vi "ramp.vi"(2 "start /single":dbl=1200.0, 3 "Number of points":i32=2, 4 "Scan type":T1(ring)=enum."Logarithmic ramp", 5 "chosen voltages":dbl[](array[numeric])=[100.0, 200.0, 300.0, 400.0, 500.0, 600.0], 6 "end":dbl=300.0) -> (0 "values":dbl[](array[numeric])=[750.0, 300.0], 1 "voltage step (linear/log)":dbl=450.0)   [LabVIEW 2018]
doc: "MeasGUI - Measurement Graphics User Interface\nCopyright (c) 2018 Frans Korhonen\n\nMeasGUI was originally developed at Institute for Atmospheric \nand Earth System Research / Physics, Faculty of Science, \nUniversity of Helsinki, Finland\n\nAssistance, experience and feedback from following persons have been \ncritical in development of MeasGUI: Michel Attoui, Juha Kangasluoma, \nLauri Ahonen, Ella Häkkinen, Markku Kulmala and Tuukka Petäjä.\n\nThis file is part of MeasGUI.\n\nThis Source Code Form is subject to the terms of the Mozilla Public\nLicense, v. 2.0. If a copy of the MPL was not distributed with this\nfile, You can obtain one at http://mozilla.org/MPL/2.0/."
panel:
  out "ramp":dbl[](graph)=[750.0, 300.0]
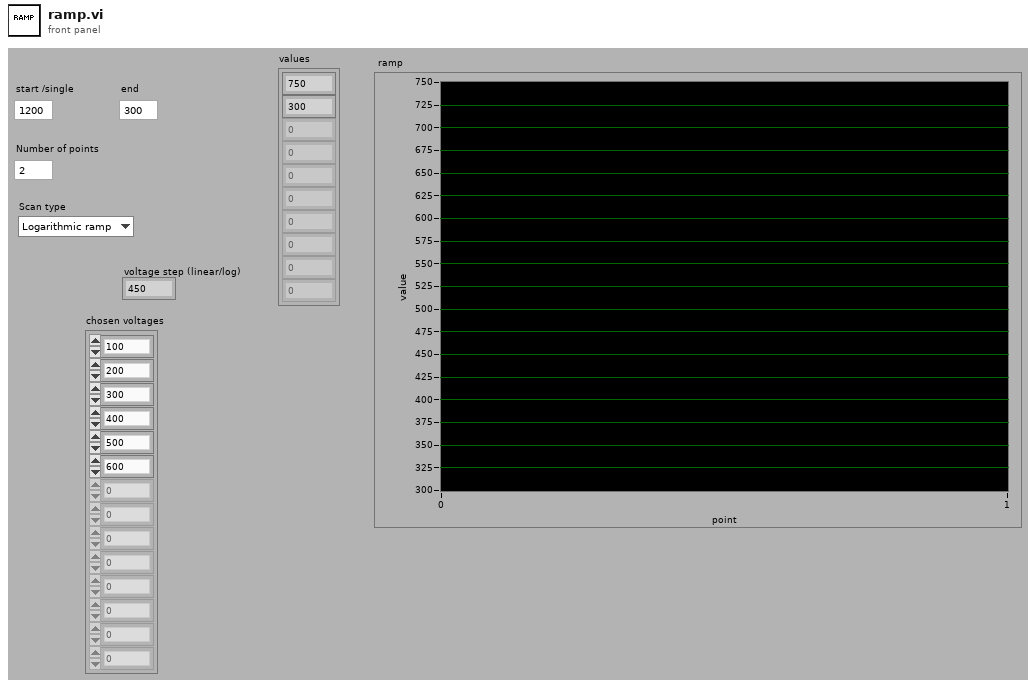
[diagram p1: front panel]
types:
  T1 = enum16{"Single", "Linear ramp", "Logarithmic ramp", "Chosen list"}
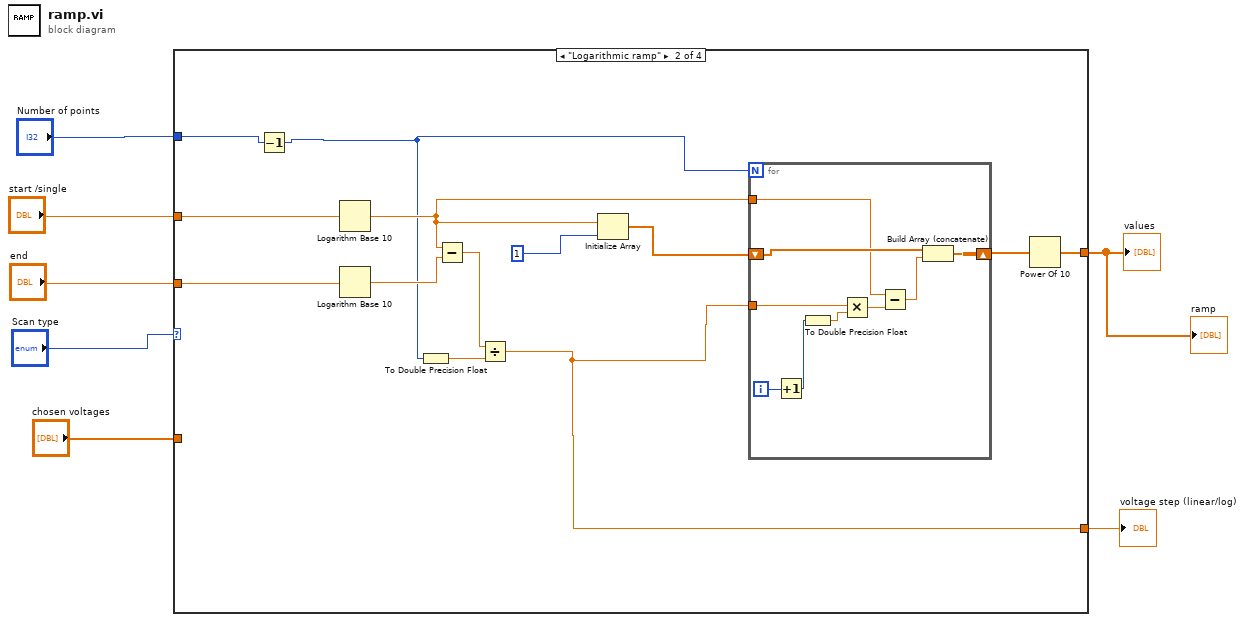
[diagram p0: block diagram]
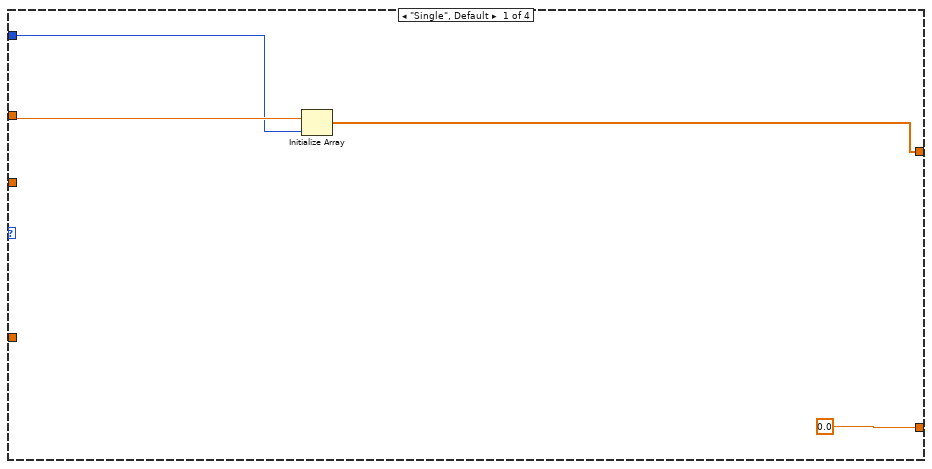
[diagram p2: hidden frame]
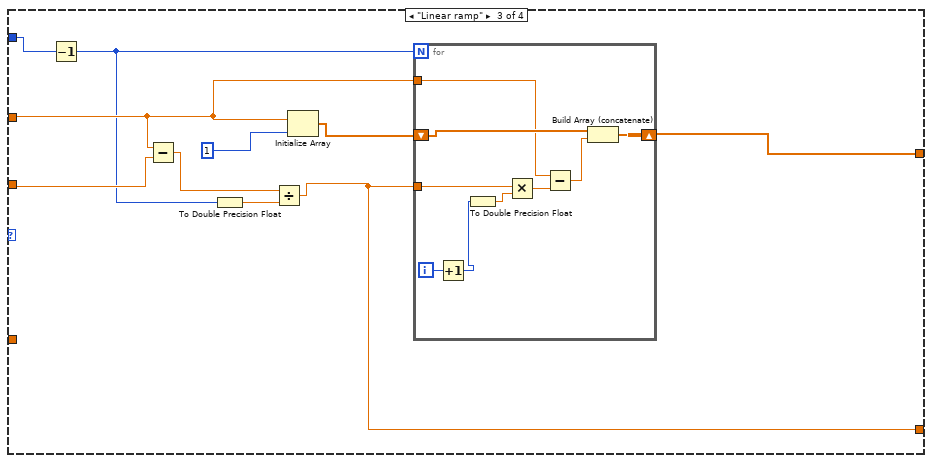
[diagram p3: hidden frame]
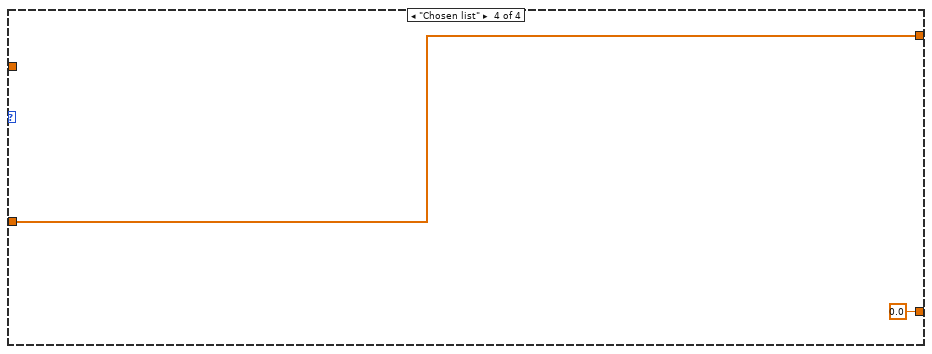
[diagram p4: hidden frame]
diagram:
  n1 = case shown="\"Logarithmic ramp\"" "Scan type" {
    tunnel: [w10 w19 w41 w54] -> w3
    tunnel: "Number of points" -> [w8 w12 w35 _]
    tunnel: "start /single" -> [w11 w16 w40 _]
    tunnel: "end" -> [_ w15 w39 _]
    tunnel: [0.0 w14 w36 0.0] -> w2
    tunnel: "chosen voltages" -> [_ _ _ w54]
    frame "Single", Default {
      n2 = Initialize Array(w11, w8) -> (w10:dbl[])
    }
    frame "Logarithmic ramp" {
      n3 = Decrement(x=w12) -> (x-1=w13:i32)
      n4 = Logarithm Base 10(1:w16) -> (0:w17:dbl)
      n5 = Logarithm Base 10(1:w15) -> (0:w22:dbl)
      n6 = To Double Precision Float(number=w13) -> (double precision float=w18:dbl)
      n7 = Subtract(x=w17, y=w22) -> (x-y=w24:dbl)
      n8 = Divide(x=w24, y=w18) -> (x/y=w14:dbl)
      n9 = Initialize Array(w17, 1) -> (w21:dbl[])
      n10 = for {
        N: w13 -> [_]
        shift-right: [w33] -> w20
        shift-left: w21 -> [w32]
        tunnel: w17 -> [w31]
        tunnel: w14 -> [w28]
        i -> [w30]
        n11 = Increment(x=w30) -> (x+1=w27:i32)
        n12 = To Double Precision Float(number=w27) -> (double precision float=w26:dbl)
        n13 = Multiply(x=w28, y=w26) -> (x*y=w29:dbl)
        n14 = Subtract(x=w31, y=w29) -> (x-y=w25:dbl)
        n15 = Build Array (concatenate)(w32, w25) -> (w33:dbl[])
      }
      n16 = Power Of 10(x=w20) -> (10^x=w19:dbl[])
    }
    frame "Linear ramp" {
      n17 = Decrement(x=w35) -> (x-1=w34:i32)
      n18 = Subtract(x=w40, y=w39) -> (x-y=w37:dbl)
      n19 = To Double Precision Float(number=w34) -> (double precision float=w38:dbl)
      n20 = Divide(x=w37, y=w38) -> (x/y=w36:dbl)
      n21 = Initialize Array(w40, 1) -> (w42:dbl[])
      n22 = for {
        N: w34 -> [_]
        shift-right: [w52] -> w41
        shift-left: w42 -> [w51]
        tunnel: w40 -> [w50]
        tunnel: w36 -> [w48]
        i -> [w45]
        n23 = Increment(x=w45) -> (x+1=w44:i32)
        n24 = To Double Precision Float(number=w44) -> (double precision float=w47:dbl)
        n25 = Multiply(x=w48, y=w47) -> (x*y=w49:dbl)
        n26 = Subtract(x=w50, y=w49) -> (x-y=w46:dbl)
        n27 = Build Array (concatenate)(w51, w46) -> (w52:dbl[])
      }
    }
    frame "Chosen list" {
    }
  }
  "values" <- w3
  "ramp" <- w3
  "voltage step (linear/log)" <- w2
